vi "Serial Port connect.vi"() -> (0 "VISA resource out":refnum<visa-resource-name>)   [LabVIEW 2017]
panel:
  out "Open/Closed":bool
  out "Link Margin":u32
  out "Channel":u32
  out "Gateway IP":string
  out "Network Mask":string
  out "Destination IP Address":string
  out "Module IP Address":string
  out "Encryption":string
  out "SSID":string
  out "Connection Status":bool
  out "Association Information (AI)":string
  in  "Open serial":bool
  in  "VISA resource name":refnum<visa-resource-name>
  # "Serial port"
  # "Network Information"
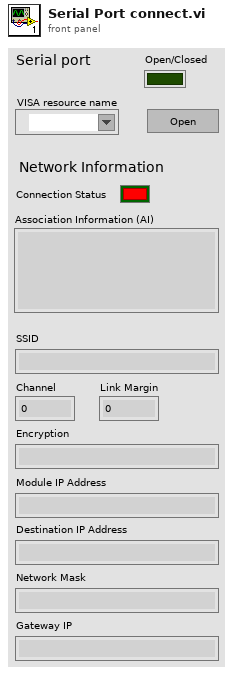
[diagram p1: front panel]
types:
  T1 = cluster{"[0]":string, "[1]":string, "[2]":string, "[3]":string, "[4]":string, "[5]":string, "[6]":string, "[7]":string, "[8]":string}
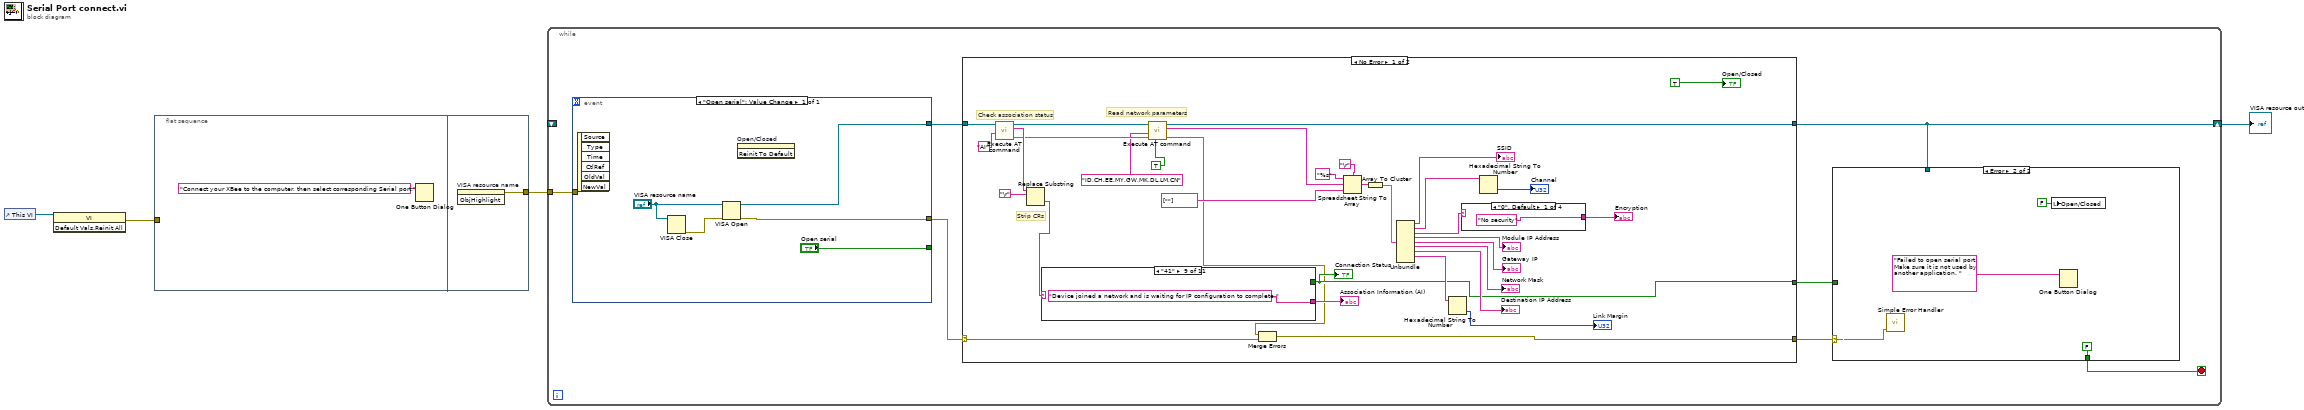
[diagram p0: block diagram]
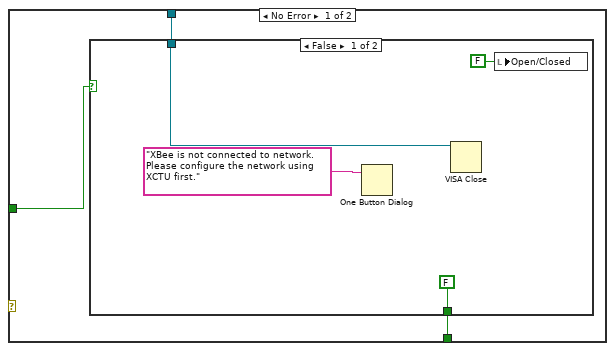
[diagram p2: hidden frame]
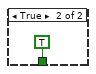
[diagram p3: hidden frame]
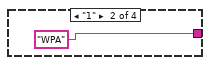
[diagram p4: hidden frame]
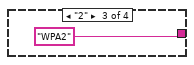
[diagram p5: hidden frame]
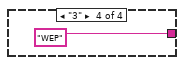
[diagram p6: hidden frame]
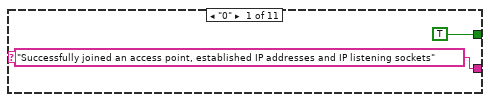
[diagram p7: hidden frame]
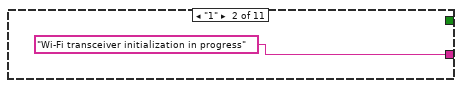
[diagram p8: hidden frame]
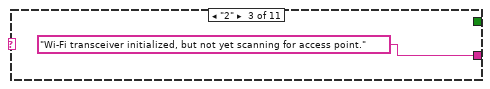
[diagram p9: hidden frame]
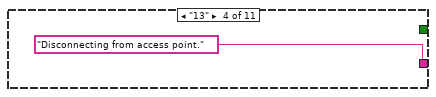
[diagram p10: hidden frame]
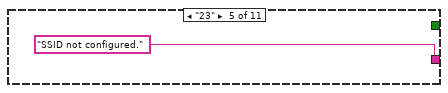
[diagram p11: hidden frame]
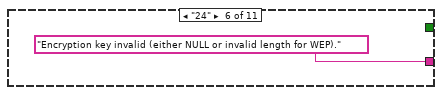
[diagram p12: hidden frame]
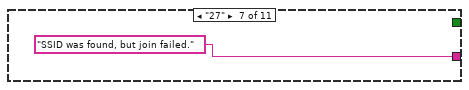
[diagram p13: hidden frame]
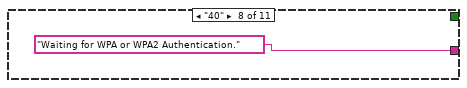
[diagram p14: hidden frame]
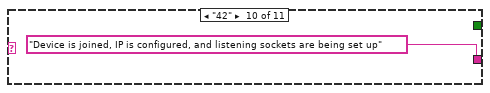
[diagram p15: hidden frame]
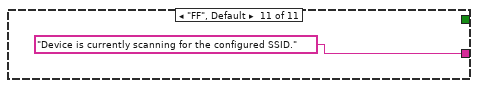
[diagram p16: hidden frame]
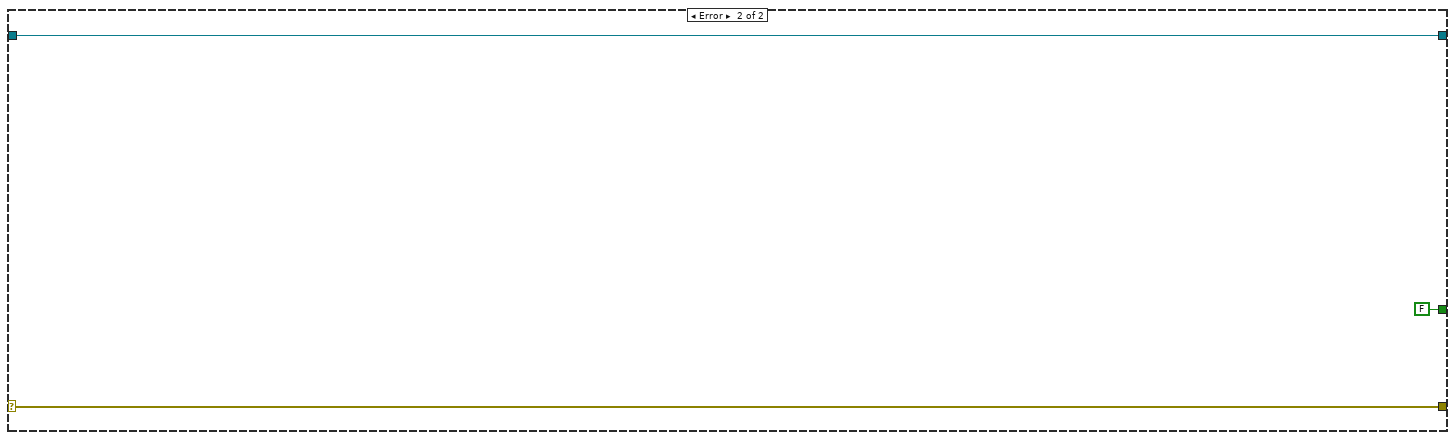
[diagram p17: hidden frame]
diagram:
  n1 = control-ref of="This VI"() -> (w4:refnum<vi>)
  n2 = invoke class="VI" method="Default Vals.Reinit All"(reference=w4) -> (error out=w3:errorcluster)  [unwired: 2 in, 2 out]
  n3 = flat-sequence {
    tunnel: w3 -> [_]
    tunnel: [w6] -> w2
    frame #0 {
      n4 = One Button Dialog(message="Connect your XBee to the computer, then select corresponding Serial port.") -> ()  [unwired: 1 in, 1 out]
    }
    frame #1 {
      n5 = invoke on="VISA resource name" class="VISAName" method="ObjHighlight"() -> (error out=w6:errorcluster)  [unwired: 3 in, 2 out]
    }
  }
  n6 = while {
    tunnel: w2 -> [w10]
    shift-right: [w7] -> w1
    shift-left: _ -> [_]
    stop <- w8 stop-if-true
    n7 = event shown="[0] \"Open serial\": Value Change" {
      selector: _ -> [_]
      dyn-events: _ -> [_]
      timeout: _ -> [_]
      tunnel: [w81] -> w12
      tunnel: [w80] -> w13
      tunnel: ["Open serial"] -> _
      tunnel: w10 -> [_]
      event "Open serial": Value Change {
        n8 = event-data() -> ()  [unwired: 1 in, 6 out]
        n9 = VISA Close(VISA resource name="VISA resource name") -> (error out=w79:errorcluster)  [unwired: 1 in]
        n10 = VISA Open(error in (no error)=w79, VISA resource name="VISA resource name") -> (VISA resource name=w81:refnum<visa-resource-name>, error out=w80:errorcluster)  [unwired: 3 in]
        n11 = invoke on="Open/Closed" class="Bool (strict)" method="Reinit To Default"() -> ()  [unwired: 3 in, 3 out]
      }
    }
    n12 = case shown="No Error" w13 {
      selector: w13 -> [w58 w77]
      tunnel: w12 -> [w45 w75]
      tunnel: [w28 w77] -> w11
      tunnel: [w31 FALSE] -> w9
      tunnel: [w26 w75] -> w7
      frame No Error {
        # "Read network parameters"
        # "Strip CRs"
        # "Check association status"
        n13 = call "Execute AT command.vi"("AT Command"="AI", "VISA resource in"=w45) -> ("error out"=w54:errorcluster, "Response message"=w56:string, "VISA resource out"=w30:refnum<visa-resource-name>)  [unwired: 6 in]
        n14 = Replace Substring(4:"\r", 5:w56) -> (0:w43:string)  [unwired: 2 in, 1 out]
        n15 = case shown="\"41\"" w43 {
          tunnel: ["Successfully joined an access point, established IP addresses and IP listening sockets" "Wi-Fi transceiver initialization in progress" "Wi-Fi transceiver initialized, but not yet scanning for access point." "Disconnecting from access point." "SSID not configured." "Encryption key invalid (either NULL or invalid length for WEP)." "SSID was found, but join failed." "Waiting for WPA or WPA2 Authentication." "Device joined a network and is waiting for IP configuration to complete." "Device is joined, IP is configured, and listening sockets are being set up" "Device is currently scanning for the configured SSID."] -> w44
          tunnel: [TRUE _ _ _ _ _ _ _ _ _ _] -> w31
          frame "0" {
          }
          frame "1" {
          }
          frame "2" {
          }
          frame "13" {
          }
          frame "23" {
          }
          frame "24" {
          }
          frame "27" {
          }
          frame "40" {
          }
          frame "41" {
          }
          frame "42" {
          }
          frame "FF", Default {
          }
        }
        "Association Information (AI)" <- w44
        "Connection Status" <- w31
        n16 = call "Execute AT command.vi"("Exit AT mode"=TRUE, "error in (no error)"=w54, "AT Command"="ID,CH,EE,MY,GW,MK,DL,LM,CN", "VISA resource in"=w30) -> ("error out"=w27:errorcluster, "Response message"=w51:string, "VISA resource out"=w26:refnum<visa-resource-name>)  [unwired: 4 in]
        n17 = Merge Errors(w27, w58) -> (w28:errorcluster)
        n18 = Spreadsheet String To Array(delimiter (Tab)="\r", format string="%s", spreadsheet string=w51, array type (2D Dbl)=string[] [""]) -> (array=w47:string[])
        n19 = Array To Cluster(array=w47) -> (cluster=w46:T1)
        n20 = Unbundle(w46) -> ("[0]"=→"SSID":string, "[1]"=w41:string, "[2]"=w39:string, "[3]"=→"Module IP Address":string, "[4]"=→"Gateway IP":string, "[5]"=→"Network Mask":string, "[6]"=→"Destination IP Address":string, "[7]"=w33:string)  [unwired: 1 out]
        n21 = Hexadecimal String To Number(string=w33) -> (number=→"Link Margin":u32)  [unwired: 2 in, 1 out]
        n22 = case shown="\"0\", Default" w39 {
          tunnel: ["No security" ("format string") "WPA" "WPA2" "WEP"] -> w38
          frame "0", Default {
          }
          frame "1" {
          }
          frame "2" {
          }
          frame "3" {
          }
        }
        "Encryption" <- w38
        n23 = Hexadecimal String To Number(string=w41) -> (number=→"Channel":u32)  [unwired: 2 in, 1 out]
        "Open/Closed" <- TRUE
      }
      frame Error {
      }
    }
    n24 = case shown="Error" w11 {
      selector: w11 -> [_ w23]
      tunnel: w9 -> [w16 _]
      tunnel: [w15 FALSE] -> w8
      tunnel: w7 -> [w14 _]
      frame No Error {
        n25 = case shown="False" w16 {
          tunnel: [FALSE TRUE] -> w15
          tunnel: w14 -> [w17 _]
          frame False {
            n26 = One Button Dialog(message="XBee is not connected to network. Please configure the network using XCTU first.") -> ()  [unwired: 1 in, 1 out]
            n27 = VISA Close(VISA resource name=w17) -> ()  [unwired: 1 in, 1 out]
            n28 = local write "Open/Closed"(FALSE ("Open/Closed")) -> ()
          }
          frame True {
          }
        }
      }
      frame Error {
        n29 = call <vilib>:"Simple Error Handler.vi"("error in (no error)"=w23) -> ()  [unwired: 4 in, 5 out]
        n30 = local write "Open/Closed"(FALSE ("Open/Closed")) -> ()
        n31 = One Button Dialog(message="Failed to open serial port. Make sure it is not used by another application. ") -> ()  [unwired: 1 in, 1 out]
      }
    }
  }
  "VISA resource out" <- w1
